vi "HXG2_HeatLoadAir_NozzleMassFlow.vi"(0 "Mdot Air (lbm/hr)":dbl, 5 "Air In Avg (°F)":dbl, 7 "Air Out Avg (°F)":dbl, 9 "RhoAir":dbl, 11 "error in (no error)":errorcluster) -> (4 "Q air (BTU/hr)":dbl, 6 "Qair (W)":dbl, 8 "CFM HX":dbl, 10 "Moist Air Cp (BTU/lb)":dbl, 15 "error out":errorcluster)   [LabVIEW 2012]
doc: "This VI will comlplete psychrometric calculations and output density of air and complete the calculation to figure out the heat load on the air side and finalizes with the conversion from SCFM to ACFM. The ACFM calculation is documented at the bottom of the block diagram."
panel:
  out "Qair Std":dbl
  out "Cp Wtr (BTU/lbm R)":dbl
  out "Cp Dry Air (BTU/lbm R)":dbl
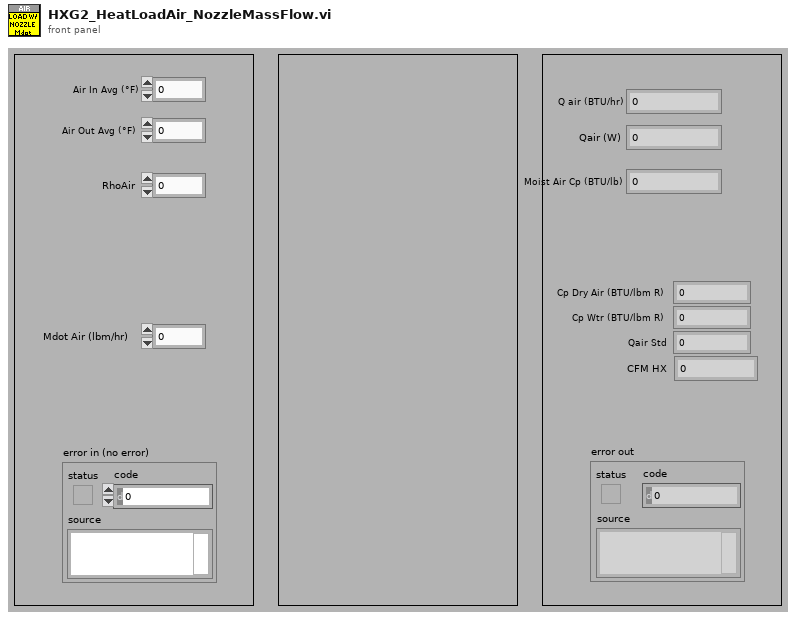
[diagram p1: front panel]
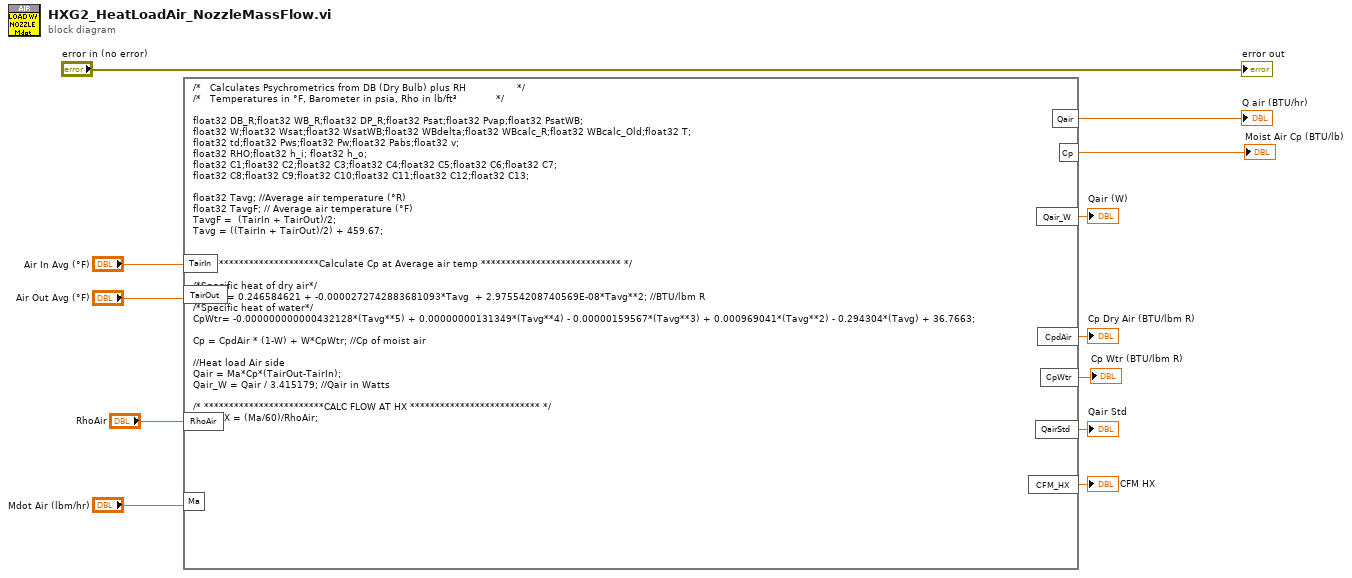
[diagram p0: block diagram]
diagram:
  n1 = formula code="/*   Calculates Psychrometrics from DB (Dry Bulb) plus RH                 */\n/*   Temperatures in °F, Barometer in psia, Rho in lb/ft³             */\n\nfloat32 DB_R;float32 WB_R;float32 DP_R;float32 Psat;float32 Pvap;float32 PsatWB;\nfloat32 W;float32 Wsat;float32 WsatWB;float32 WBdelta;float32 WBcalc_R;float32 WBcalc_Old;float32 T;\nfloat32 td;float32 Pws;float32 Pw;float32 Pabs;float32 v;\nfloat32 RHO;float32 h_i; float32 h_o;\nfloat32 C1;float32 C2;float32 C3;float32 C4;float32 C5;float32 C6;float32 C7;\nfloat32 C8;float32 C9;float32 C10;float32 C11;float32 C12;float32 C13;\n\nfloat32 Tavg; //Average air temperature (°R)\nfloat32 TavgF; // Average air temperature (°F)\nTavgF =  (TairIn + TairOut)/2;\nTavg = ((TairIn + TairOut)/2) + 459.67;\n\n\n/* ***********************Calculate Cp at Average air temp **************************** */\n\n/*Specific heat of dry air*/\nCpdAir = 0.246584621 + -0.0000272742883681093*Tavg  + 2.97554208740569E-08*Tavg**2; //BTU/lbm R\n/*Specific heat of water*/\nCpWtr= -0.000000000000432128*(Tavg**5) + 0.00000000131349*(Tavg**4) - 0.00000159567*(Tavg**3) + 0.000969041*(Tavg**2) - 0.294304*(Tavg) + 36.7663;\n\nCp = CpdAir * (1-W) + W*CpWtr; //Cp of moist air\n\n//Heat load Air side\nQair = Ma*Cp*(TairOut-TairIn);\nQair_W = Qair / 3.415179; //Qair in Watts\n\n/* ************************CALC FLOW AT HX ************************** */\nCFM_HX = (Ma/60)/RhoAir;"("TairIn"="Air In Avg (°F)", "TairOut"="Air Out Avg (°F)", "Ma"="Mdot Air (lbm/hr)", "RhoAir"="RhoAir") -> ("Qair"=→"Q air (BTU/hr)":dbl, "Cp"=→"Moist Air Cp (BTU/lb)":dbl, "Qair_W"=→"Qair (W)":dbl, "CpdAir"=→"Cp Dry Air (BTU/lbm R)":dbl, "CpWtr"=→"Cp Wtr (BTU/lbm R)":dbl, "QairStd"=→"Qair Std":dbl, "CFM_HX"=→"CFM HX":dbl)
  "error out" <- "error in (no error)"
